vi "Update.vi"(8 "error in":errorcluster, 10 "NewData":refnum<class "Data.lvclass">, 11 "Data Subject in":refnum<class "Publisher.lvclass">) -> (0 "error out":errorcluster, 3 "Data Subject out":refnum<class "Publisher.lvclass">)   [LabVIEW 2014, in "Publisher.lvclass"]
doc: "Let all subscribers know that there is data on the line."
uses:
  Publisher.lvclass
  Data/Data.lvclass
  Publisher.lvclass/Publisher.ctl
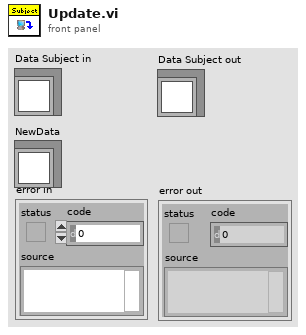
[diagram p1: front panel]
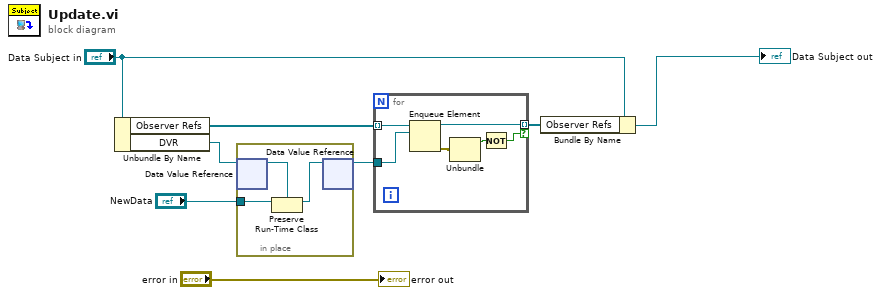
[diagram p0: block diagram]
diagram:
  n1 = Unbundle By Name("Data Subject in") -> ("Observer Refs"=w7:refnum<queue>[], "DVR"=w2:refnum<data-value>)
  n2 = in-place {
    in-place-border: "NewData" -> [w10]
    n3 = in-place-dvr #1(w2) -> (w11:refnum<class "Data.lvclass">)  [unwired: 1 out]
    n4 = Preserve Run-Time Class(object in=w10, 2:w11) -> (object out=w9:refnum<class "Data.lvclass">)  [unwired: 1 in, 1 out]
    n5 = in-place-dvr #1(w9) -> (w1:refnum<data-value>)  [unwired: 1 out]
  }
  n6 = for {
    tunnel: w7 -> [w17] mode=indexing
    tunnel: w1 -> [w16]
    tunnel: [w15] -> w6 mode=indexing if=w12
    n7 = Enqueue Element(queue=w17, element=w16) -> (queue out=w15:refnum<queue>, error out=w14:errorcluster)  [unwired: 2 in, 1 out]
    n8 = Unbundle(w14) -> ("status"=w13:bool)  [unwired: 2 out]
    n9 = Not(x=w13) -> (.not. x?=w12:bool)
  }
  n10 = Bundle By Name(cluster="Data Subject in", "Observer Refs"=w6) -> (→"Data Subject out":refnum<class "Publisher.lvclass">)
  "error out" <- "error in"
